vi "运维调试_采配水.vi"() -> ()   [LabVIEW 2016, in "PLC.lvlib"]
uses:
  PLC.lvlib
  <vilib>/Plasmionique/MB Master/MB_Master/MB_Master.lvclass
  <vilib>/Utility/miscctls.llb/LVPointTypeDef.ctl
  <vilib>/Plasmionique/MB Master/MB_Master_TCP/MB_Master_TCP.lvclass
  D:/Program Files (x86)/National Instruments/LabVIEW 2016/vi.lib/Plasmionique/MB Master/MB_Master/MB_Master.lvclass
  <vilib>/NI/Modbus Library/API/Wrapper/Create TCP Slave.vi
  <vilib>/NI/Modbus Library/API/slave/Modbus Slave.lvclass
  <vilib>/Plasmionique/MB Master/MB Master.lvlib
  <vilib>/NI/Modbus Library/API/Wrapper/API Main.lvlib
panel:
  out "R116":i16 caption="储水时间设定"
  out "R115":i16 caption="清洗频次设定"
  out "R114":i16 caption="排液时间"
  out "R113":i16 caption="沉淀池清洗时间"
  out "R112":i16 caption="流通池清洗时间"
  out "R111":i16 caption="吹气时间"
  out "R110":i16 caption="外部管路清洗时间"
  out "R109":i16 caption="配水时间"
  out "R108":i16 caption="沉淀时间"
  out "R107":i16 caption="液位开关报警时间"
  out "R106":i16 caption="进样超时时间"
  out "R105":i16 caption="沉淀池润洗时间"
  out "R104":i16 caption="流通池润洗时间"
  out "沉淀池进样阀计时":dbl
  out "流通池进样阀计时":dbl
  in  "V3-R":bool
  in  "V3-G":bool
  out "状态":u16[](array[numeric])
  in  "更新程序":bool
  out "清洗次数":u16
  out "当前启动泵号":u16(ring) items=["1号泵", "2号泵"]
  in  "R117":u16(ring) caption="水箱储水水体" items=["自来水", "水样"]
  out "增压泵计时":dbl
  out "M2工作计时":dbl
  out "M1工作计时":dbl
  out "泵2反冲洗阀计时":dbl
  out "泵1反冲洗阀计时":dbl
  out "自来水出水阀计时":dbl
  out "进气阀计时":dbl
  out "流通池排液阀计时":dbl
  out "沉淀池排液阀计时":dbl
  out "沉淀池反冲洗阀计时":dbl
  out "流通池反冲洗阀计时":dbl
  out "泵2进样阀计时":dbl
  out "泵1进样阀计时":dbl
  in  "M3":bool
  in  "V11":bool
  in  "V10":bool
  in  "V2":bool
  in  "V1":bool
  in  "V7":bool
  in  "V6":bool
  out "X2":bool caption="X1"
  out "采配水版本号":string
  out "通讯故障":bool
  in  "R102":u16(ring) caption="采水泵工作模式" items=["泵1单泵单管路", "泵2单泵单管路", "双泵双管路"]
  out "X7":bool caption="烟雾报警_YW"
  out "X6":bool caption="泵2过载报警_KM2"
  out "X5":bool caption="泵1过载报警_KM1"
  out "X4":bool caption="外部电源断电报警_DD1"
  out "X3":bool caption="水浸报警_SJ"
  out "X1":bool
  out "X0":bool caption="流通池液位开关_YE1"
  out "集成报警信息":string
  out "R2":i16
  out "R1":i16
  out "多列列表框":i32(listbox)
  in  "V4":bool
  in  "V5":bool
  in  "V9":bool
  in  "V8":bool
  in  "M2":bool
  in  "M1":bool
  in  "返回":bool
  in  "参数设置":bool
  in  "单步启动":bool
  in  "启动":bool
  in  "停止":bool
  # "流程计时："
  # "s"
  # "沉淀池液位开关_YE2"
  # "进样水流开关_JY"
  # "S"
  # "次"
  # "S"
  # "S"
  # "S"
  # "S"
  # "S"
  # "S"
  # "S"
  # "S"
  # "S"
  # "S"
  # "S"
  # "单步计时："
  # "s"
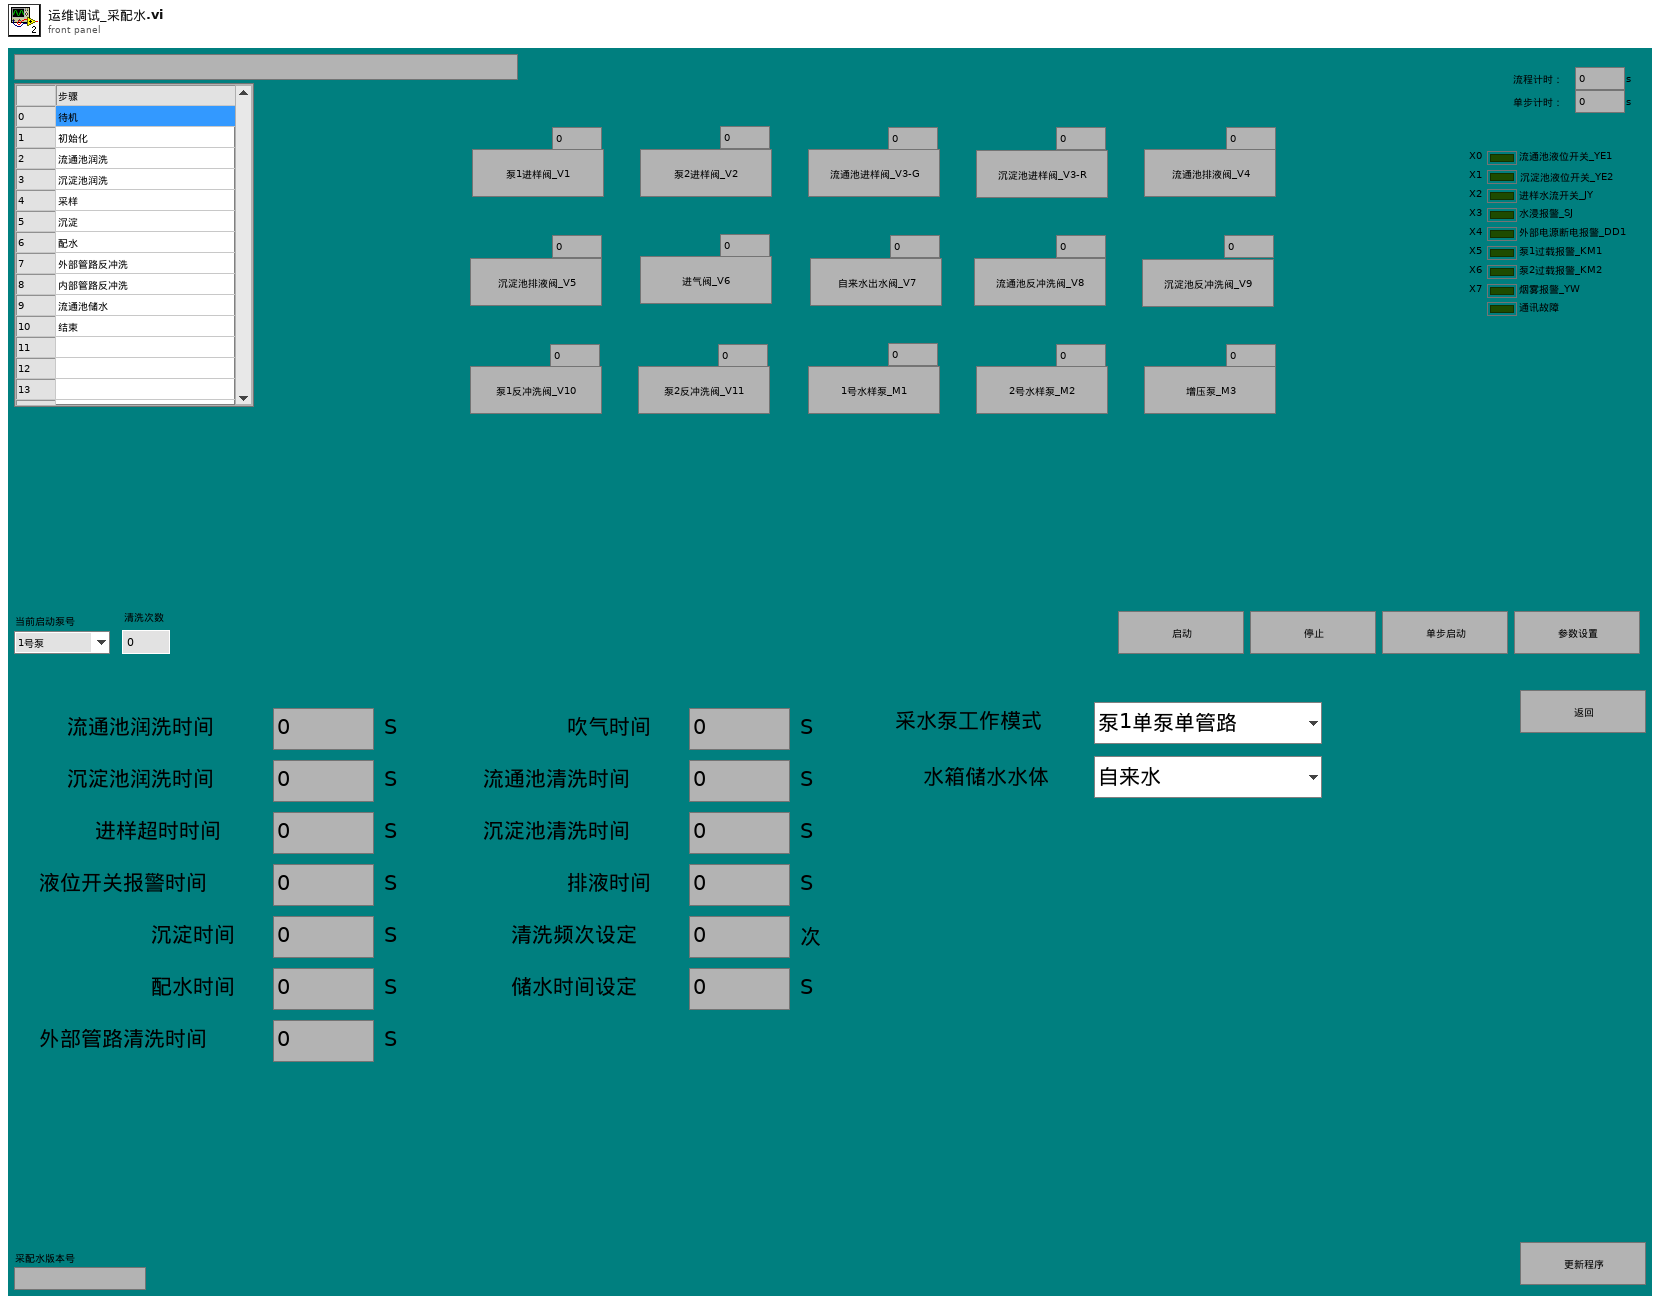
[diagram p1: front panel]
types:
  T1 = cluster{"R100":i16, "R101":i16, "R102":i16, "R103":i16, "R104":i16, "R105":i16, "R106":i16, "R107":i16, "R108":i16, "R109":i16, "R110":i16, "R111":i16, "R112":i16, "R113":i16, "R114":i16, "R115":i16, "R116":i16, "R117":i16, "R118":i16, "R119":i16}
  T2 = cluster{"R200":i16, "R201":i16, "R20 2":i16, "R20 3":i16, "R20 4":i16, "R20 5":i16, "R20 6":i16, "R20 7":i16, "R20 8":i16, "R20 9":i16, "R210":i16, "R211":i16, "R21 2":i16, "R21 3":i16, "R21 4":i16, "R21 5":i16, "R21 6":i16, "R21 7":i16, "R21 8":i16, "R21 9":i16, "R220":i16, "R221":i16, "R22 2":i16, "R22 3":i16}
  T3 = typedef "LVPointTypeDef.ctl" = cluster{"Horizontal":i16, "Vertical":i16}
  T4 = cluster{"时间标识":timestamp, "设备":string, "日志信息":string}
  T5 = cluster{"R0":i16, "R1":i16, "R2":i16, "R3":i16, "R4":i16, "R5":i16, "R6":i16, "R7":i16, "R8":i16, "R9":i16, "R10":i16, "R11":i16, "R12":i16, "R13":i16, "R14":i16, "R15":i16, "R16":i16, "R17":i16, "R18":i16, "R19":i16, "R20":i16, "R21":i16, "R22":i16, "R23":i16, "R24":i16, "R25":i16, "R26":i16, "R27":i16, "R28":i16, "R29":i16, "R30":i16, "R31":i16, "R32":i16, "R33":i16, "R34":i16, "R35":i16, "R36":i16, "R37":i16, "R38":i16, "R39":i16}
  T6 = cluster{"seconds since 1Jan1904":timestamp, "table输入":string, string, "table输入":string}
  T7 = cluster{"时间标识":timestamp, "设备":string, "日志信息":string, "流程参数":string}
  T8 = cluster{"命令":string, cluster{"starting address":u16, "holding register value":u16}}
  T9 = cluster{"命令":string, "数据":cluster{"starting address":u16, "holding register value":u16}}
  T10 = cluster{"命令":string, "数据":cluster{"starting address":u16, "holding register values":u16[]}}
  T11 = cluster{"命令":string, "data":cluster{"starting address":u16, "coil values":bool[]}}
  T12 = cluster{"测试模式":enum16{"正常测试", "集成干预"}, "参数启用":cluster{"氨氮":bool, "总磷":bool, "总氮":bool, "多参数":bool, "CODMn":bool, "CODcr":bool}}
  T13 = enum32{"Bad", "Idle", "Run top level", "Running"}
  T14 = cluster{"starting address":u16, "holding register values":u16[]}
  T15 = cluster{"starting address":u16, "holding register value":u16}
  T16 = cluster{"starting address":u16, "coil values":bool[]}
  T17 = cluster{"Registers[0]":u16, "Registers[1]":u16, "Registers[2]":u16, "Registers[3]":u16, "Registers[4]":u16, "Registers[5]":u16, "Registers[6]":u16, "Registers[7]":u16, "Registers[8]":u16, "Registers[9]":u16, "Registers[10]":u16, "Registers[11]":u16, "Registers[12]":u16, "Registers[13]":u16, "Registers[14]":u16, "Registers[15]":u16, "Registers[16]":u16, "Registers[17]":u16, "Registers[18]":u16, "Registers[19]":u16, "Registers[20]":u16, "Registers[21]":u16, "Registers[22]":u16, "Registers[23]":u16, "Registers[24]":u16, "Registers[25]":u16, "Registers[26]":u16, "Registers[27]":u16, "Registers[28]":u16, "Registers[29]":u16, "Registers[30]":u16, "Registers[31]":u16, "Registers[32]":u16, "Registers[33]":u16, "Registers[34]":u16, "Registers[35]":u16, "Registers[36]":u16, "Registers[37]":u16, "Registers[38]":u16, "Registers[39]":u16}
  T18 = cluster{"Registers[0]":u16, "Registers[1]":u16, "Registers[2]":u16, "Registers[3]":u16, "Registers[4]":u16, "Registers[5]":u16, "Registers[6]":u16, "Registers[7]":u16, "Registers[8]":u16, "Registers[9]":u16, "Registers[10]":u16, "Registers[11]":u16, "Registers[12]":u16, "Registers[13]":u16, "Registers[14]":u16, "Registers[15]":u16, "Registers[16]":u16, "Registers[17]":u16, "Registers[18]":u16, "Registers[19]":u16, "Registers[20]":u16, "Registers[21]":u16, "Registers[22]":u16, "Registers[23]":u16}
  T19 = cluster{"Registers[0]":u16, "Registers[1]":u16, "Registers[2]":u16, "Registers[3]":u16, "Registers[4]":u16, "Registers[5]":u16}
  T20 = cluster{"Registers[0]":u16, "Registers[1]":u16, "Registers[2]":u16, "Registers[3]":u16, "Registers[4]":u16, "Registers[5]":u16, "Registers[6]":u16, "Registers[7]":u16, "Registers[8]":u16, "Registers[9]":u16, "Registers[10]":u16, "Registers[11]":u16, "Registers[12]":u16, "Registers[13]":u16, "Registers[14]":u16, "Registers[15]":u16, "Registers[16]":u16, "Registers[17]":u16, "Registers[18]":u16, "Registers[19]":u16}
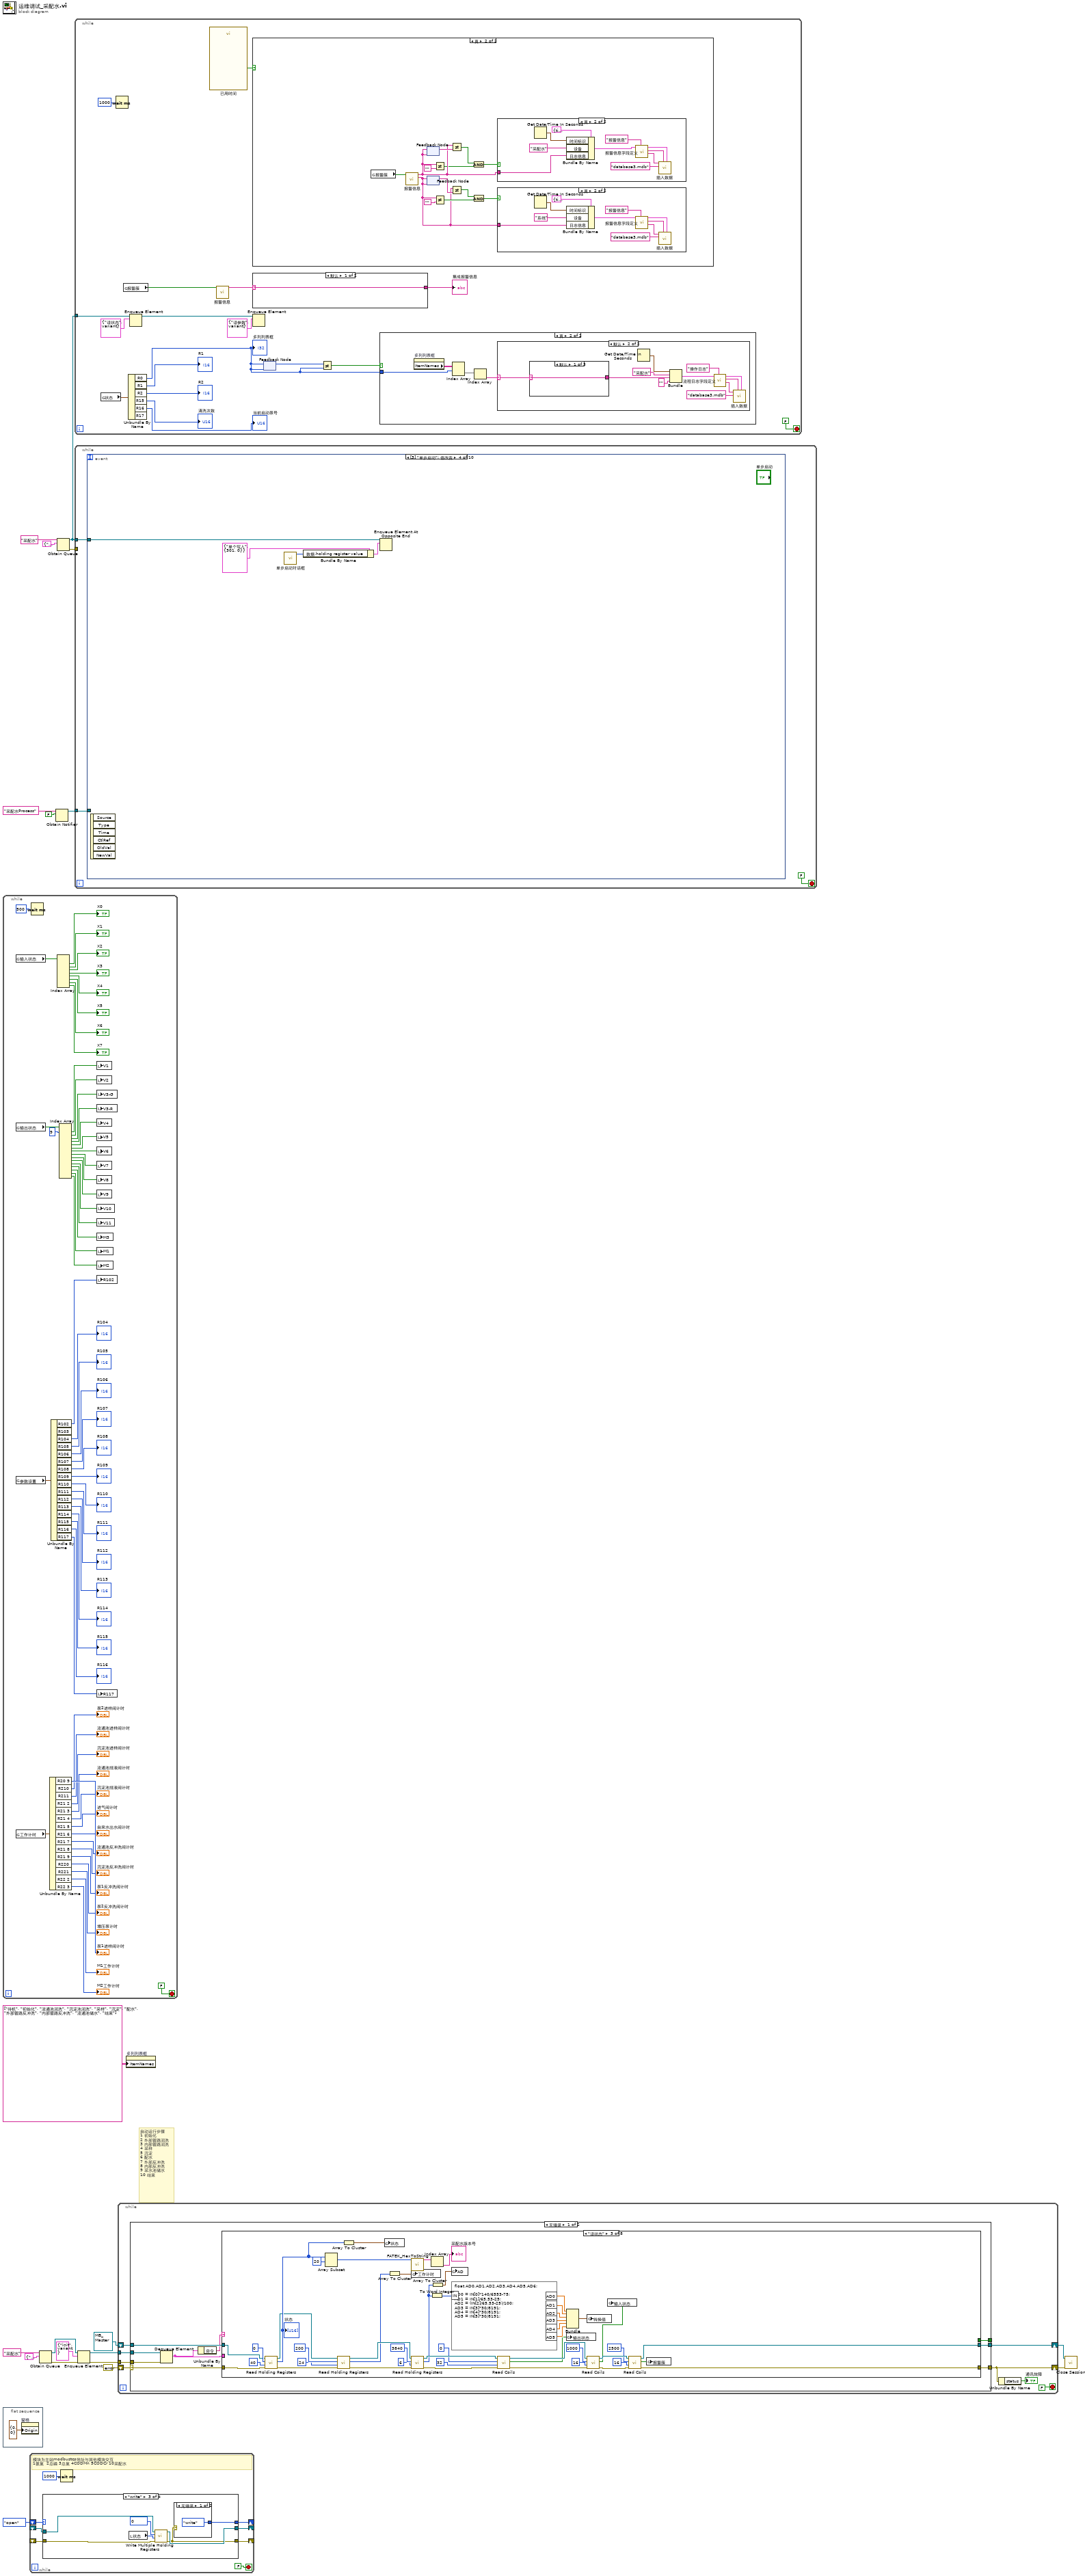
[diagram p0: block diagram]
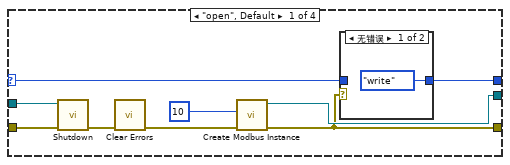
[diagram p2: hidden frame]
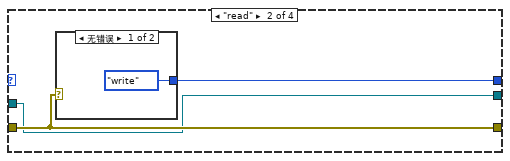
[diagram p4: hidden frame]
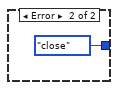
[diagram p5: hidden frame]
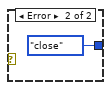
[diagram p6: hidden frame]
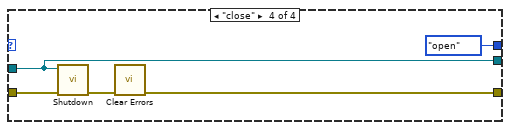
[diagram p7: hidden frame]
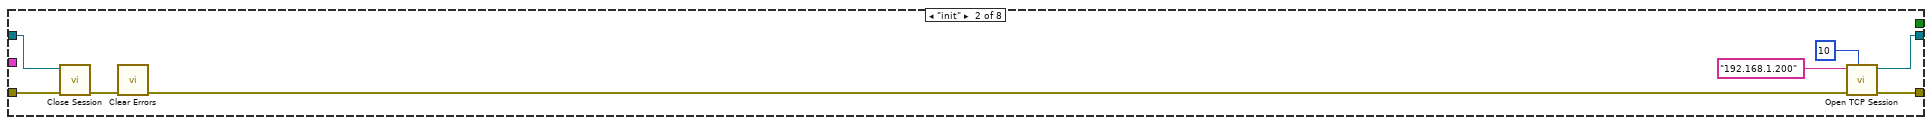
[diagram p9: hidden frame]
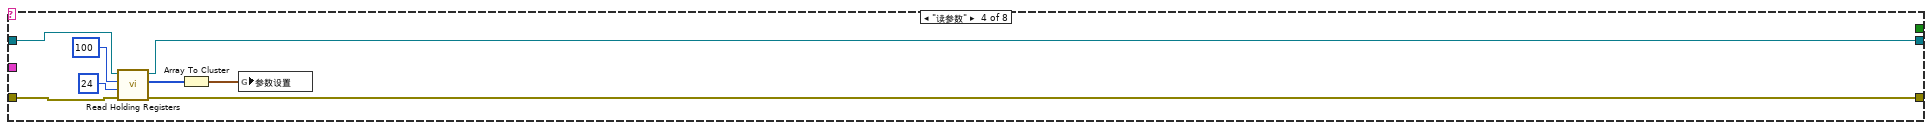
[diagram p10: hidden frame]
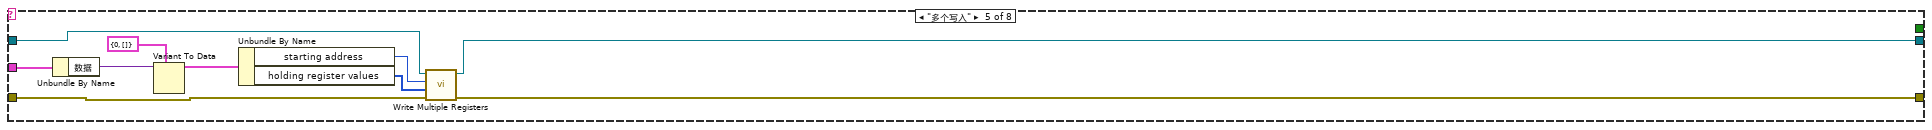
[diagram p11: hidden frame]
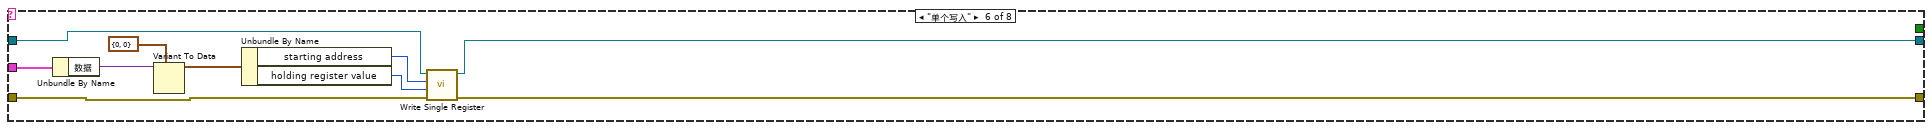
[diagram p12: hidden frame]
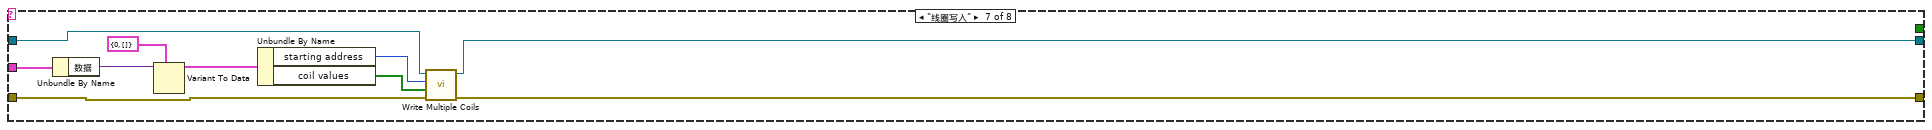
[diagram p13: hidden frame]
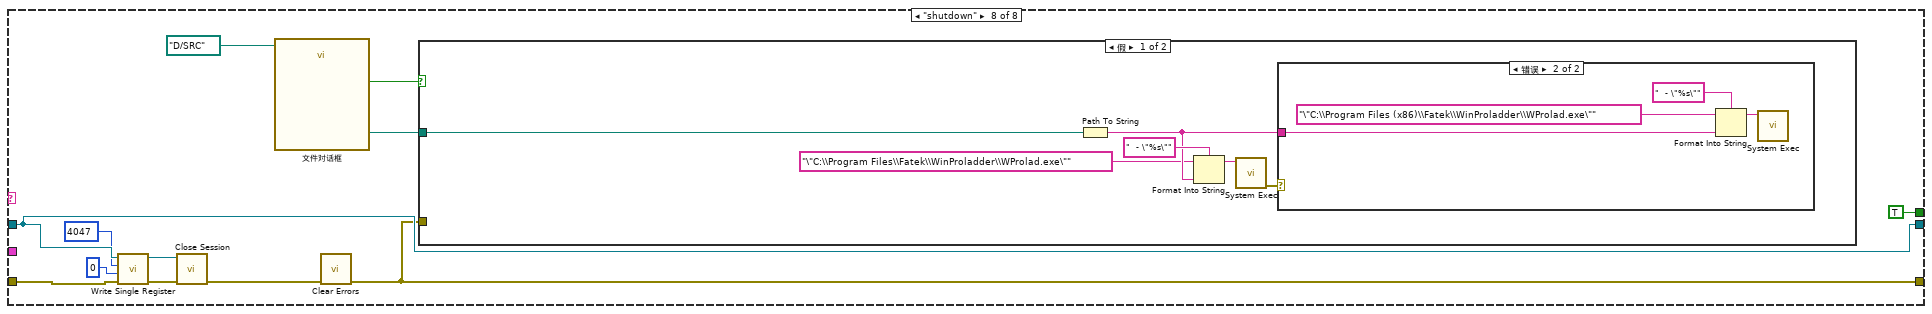
[diagram p14: hidden frame]
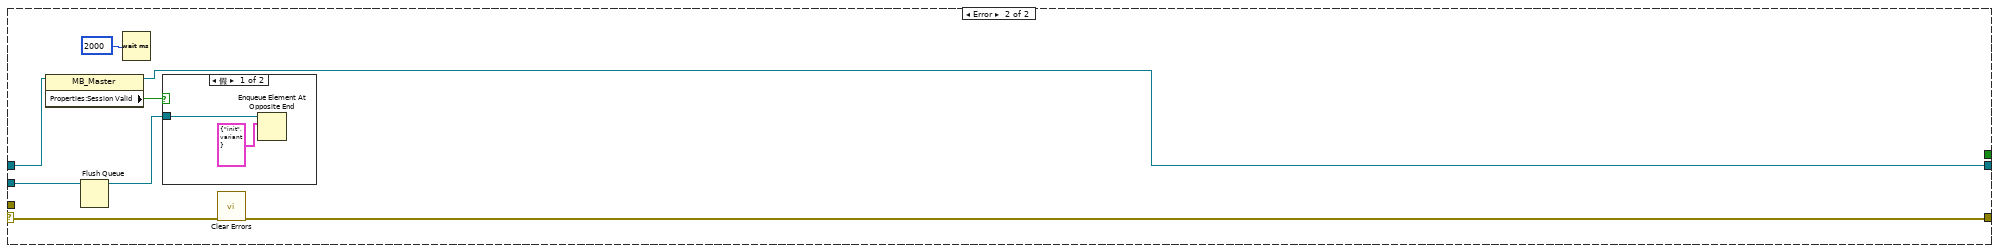
[diagram p17: hidden frame]
diagram:
  # "自动运行步骤\n1 初始化\n2 外部管路润洗\n3 内部管路润洗\n4 采样\n5 沉淀\n6 配水\n7 外部反冲洗\n8 内部反冲洗\n9 采水池储水\n10 结束"
  n1 = while {
    stop <- FALSE stop-if-true
    n2 = global read "采配水全局变量.vi" "输入状态"() -> (w63:bool[])
    n3 = global read "采配水全局变量.vi" "输出状态"() -> (w79:bool[])
    n4 = global read "采配水全局变量.vi" "参数设置"() -> (w36:T1)
    n5 = global read "采配水全局变量.vi" "工作计时"() -> (w52:T2)
    n6 = Wait (ms)(milliseconds to wait=u32 500 ("等待时间（毫秒）")) -> ()  [unwired: 1 out]
    n7 = Unbundle By Name(w52) -> ("R20 9"=→"泵1进样阀计时":i16, "R210"=→"泵2进样阀计时":i16, "R211"=→"流通池进样阀计时":i16, "R21 2"=→"沉淀池进样阀计时":i16, "R21 3"=→"流通池排液阀计时":i16, "R21 4"=→"沉淀池排液阀计时":i16, "R21 5"=→"进气阀计时":i16, "R21 6"=→"自来水出水阀计时":i16, "R21 7"=→"流通池反冲洗阀计时":i16, "R21 8"=→"沉淀池反冲洗阀计时":i16, "R21 9"=→"泵1反冲洗阀计时":i16, "R220"=→"泵2反冲洗阀计时":i16, "R221"=→"增压泵计时":i16, "R22 2"=→"M1工作计时":i16, "R22 3"=→"M2工作计时":i16)
    n8 = Unbundle By Name(w36) -> ("R102"=w35:i16, "R104"=→"R104":i16, "R105"=→"R105":i16, "R106"=→"R106":i16, "R107"=→"R107":i16, "R108"=→"R108":i16, "R109"=→"R109":i16, "R110"=→"R110":i16, "R111"=→"R111":i16, "R112"=→"R112":i16, "R113"=→"R113":i16, "R114"=→"R114":i16, "R115"=→"R115":i16, "R116"=→"R116":i16, "R117"=w21:i16)  [unwired: 1 out]
    n9 = Index Array(array=w63) -> (element #1=→"X0":bool, element #2=→"X1":bool, element #3=→"X2":bool, element #4=→"X3":bool, element #5=→"X4":bool, element #6=→"X5":bool, element #7=→"X6":bool, element #8=→"X7":bool)  [unwired: 8 in]
    n10 = Index Array(array=w79, index #1=9 ("索引")) -> (element #1=w77:bool, element #2=w76:bool, element #3=w75:bool, element #4=w74:bool, element #5=w73:bool, element #6=w72:bool, element #7=w71:bool, element #8=w70:bool, element #9=w53:bool, element #10=w54:bool, element #11=w69:bool, element #12=w68:bool, element #13=w67:bool, element #14=w66:bool, element #15=w65:bool)  [unwired: 14 in]
    n11 = local write "V1"(w77) -> ()
    n12 = local write "V2"(w76) -> ()
    n13 = local write "V3-G"(w75) -> ()
    n14 = local write "V3-R"(w74) -> ()
    n15 = local write "V4"(w73) -> ()
    n16 = local write "V5"(w72) -> ()
    n17 = local write "V6"(w71) -> ()
    n18 = local write "V7"(w70) -> ()
    n19 = local write "V8"(w53) -> ()
    n20 = local write "V9"(w54) -> ()
    n21 = local write "V10"(w69) -> ()
    n22 = local write "V11"(w68) -> ()
    n23 = local write "M3"(w67) -> ()
    n24 = local write "M1"(w66) -> ()
    n25 = local write "M2"(w65) -> ()
    n26 = local write "R102"(w35) -> ()
    n27 = local write "R117"(w21) -> ()
  }
  n28 = flat-sequence {
    frame #0 {
      n29 = property on="窗格" class="Pane"("Origin"=T3 {"Horizontal"=0, "Vertical"=0} ("原点")) -> ()  [unwired: 2 in, 2 out]
    }
  }
  n30 = while {
    shift-right: [w87] -> _
    shift-left: _ -> [w89]
    shift-right: [w86] -> _
    shift-left: _ -> [w88]
    shift-right: [w83] -> _
    shift-left: enum16{"open", "read", "write", "close"}."open" -> [w84]
    stop <- FALSE stop-if-true
    # "模块为主站modbustcp地址与其他模块交互\n1氨氮  2总磷 3总氮 4CODMn 5CODCr 10采配水"
    n31 = case shown="\"write\"" w84 {
      selector: w84 -> [w98 _ _ _]
      tunnel: w89 -> [w92 w101 w111 w117]
      tunnel: w88 -> [w91 w102 w110 w116]
      tunnel: [w95 w101 w108 w117] -> w87
      tunnel: [w94 w102 w107 w119] -> w86
      tunnel: [w97 w103 w112 enum16{"open", "read", "write", "close"}."open"] -> w83
      frame "open", Default {
        n32 = call-dynamic "Shutdown.vi"("error in"=w91, "Modbus slave in"=w92) -> ("error out"=w90:errorcluster)  [unwired: 9 in]
        n33 = call <vilib>:"Clear Errors.vi"("error in (no error)"=w90) -> ("error out"=w93:errorcluster)  [unwired: 5 in, 1 out]
        n34 = call-poly <vilib>:"Create Modbus Instance.vi"("error in"=w93, "port (502)"=u16 10) -> ("error out"=w94:errorcluster, "TCP slave instance"=w95:refnum<class "Modbus Slave.lvclass">)  [unwired: 8 in]
        n35 = case shown="无错误" w94 {
          tunnel: w98 -> [_ w100]
          tunnel: [enum16{"open", "read", "write", "close"}."write" w100] -> w97
          frame No Error {
          }
          frame Error {
          }
        }
      }
      frame "read" {
        n36 = case shown="无错误" w102 {
          tunnel: [enum16{"open", "read", "write", "close"}."write" enum16{"open", "read", "write", "close"}."close"] -> w103
          frame No Error {
          }
          frame Error {
          }
        }
      }
      frame "write" {
        n37 = local read "状态"() -> (w106:u16[])
        n38 = call-dynamic "Write Multiple Holding Registers.vi"("error in"=w110, "registers to write"=w106, "starting address"=u16 0, "Modbus slave in"=w111) -> ("error out"=w107:errorcluster, "Modbus slave out"=w108:refnum<class "Modbus Slave.lvclass">)  [unwired: 6 in]
        n39 = case shown="无错误" w107 {
          tunnel: [enum16{"open", "read", "write", "close"}."write" enum16{"open", "read", "write", "close"}."close"] -> w112
          frame No Error {
          }
          frame Error {
          }
        }
      }
      frame "close" {
        n40 = call-dynamic "Shutdown.vi"("error in"=w116, "Modbus slave in"=w117) -> ("error out"=w115:errorcluster)  [unwired: 9 in]
        n41 = call <vilib>:"Clear Errors.vi"("error in (no error)"=w115) -> ("error out"=w119:errorcluster)  [unwired: 5 in, 1 out]
      }
    }
    n42 = Wait (ms)(milliseconds to wait=u32 1000 ("等待时间（毫秒）")) -> ()  [unwired: 1 out]
  }
  n43 = Obtain Queue(name (unnamed)="采配水" ("名称（未命名）"), element data type=cluster{"命令":string, "数据":variant} {"命令"="", "数据"=variant}) -> (queue out=w10:refnum<queue>, error out=w9:errorcluster)  [unwired: 3 in, 1 out]
  n44 = Obtain Notifier(name (unnamed)="采配水Process" ("名称（未命名）"), notification data type=FALSE) -> (notifier out=w13:refnum<notifier>)  [unwired: 2 in, 2 out]
  n45 = Obtain Queue(name (unnamed)="采配水" ("名称（未命名）"), element data type=cluster{"命令":string, "数据":variant} {"命令"="", "数据"=variant}) -> (queue out=w17:refnum<queue>, error out=w18:errorcluster)  [unwired: 3 in, 1 out]
  n46 = while {
    tunnel: w17 -> [w136]
    stop <- FALSE stop-if-true
    n47 = global read "采配水全局变量.vi" "状态"() -> (w134:T5)
    n48 = Wait (ms)(milliseconds to wait=u32 1000 ("等待时间（毫秒）")) -> ()  [unwired: 1 out]
    n49 = global read "采配水全局变量.vi" "报警簇"() -> (w130:bool[])
    n50 = Unbundle By Name(w134) -> ("R0"=w123:i16, "R1"=→"R1":i16, "R2"=→"R2":i16, "R15"=→"清洗次数":i16, "R16"=→"当前启动泵号":i16)  [unwired: 1 out]
    "多列列表框" <- w123
    n51 = Enqueue Element(queue=w136, element=cluster{"命令":string, "数据":variant} {"命令"="读状态", "数据"=variant} ("元素")) -> (queue out=w125:refnum<queue>)  [unwired: 2 in, 2 out]
    n52 = call "已用时间"() -> ("Time has Elapsed"=w128:bool)  [unwired: 12 in, 7 out]
    n53 = call "报警信息.vi"("报警簇"=w130) -> ("采配水报警信息"=w122:string)  [unwired: 9 in, 1 out]
    n54 = case shown="真" w128 {
      frame False {
      }
      frame True {
        n55 = global read "采配水全局变量.vi" "报警簇"() -> (w150:bool[])
        n56 = call "报警信息.vi"("报警簇"=w150) -> ("系统报警信息"=w139:string, "采配水报警信息"=w146:string)  [unwired: 9 in]
        n57 = feedback #1(w146) -> (w149:string)
        n58 = feedback-in #1(w146) -> ()
        n59 = feedback #2(w139) -> (w140:string)
        n60 = feedback-in #2(w139) -> ()
        n61 = Not Equal?(x=w146, y="") -> (x != y?=w144:bool)
        n62 = Not Equal?(x=w139, y="") -> (x != y?=w143:bool)
        n63 = Not Equal?(x=w146, y=w149) -> (x != y?=w148:bool)
        n64 = Not Equal?(x=w139, y=w140) -> (x != y?=w141:bool)
        n65 = And(x=w148, y=w144) -> (x .and. y?=w147:bool)
        n66 = And(x=w141, y=w143) -> (x .and. y?=w138:bool)
        n67 = case shown="真" w147 {
          tunnel: w146 -> [_ w161]
          frame False {
          }
          frame True {
            n68 = Get Date/Time In Seconds() -> (seconds since 1Jan1904=w163:timestamp)
            n69 = Bundle By Name(cluster=T4 {"时间标识"=timestamp(0 s since 1904-01-01), "设备"="", "日志信息"=""} ("data in"), "时间标识"=w163, "设备"="采配水", "日志信息"=w161) -> (w164:T4)
            n70 = call "报警信息字段定义.vi"("table输入"="报警信息", "data in"=w164) -> ("table输出"=w168:string, "columns"=w169:string[], "data out"=w170:T4)  [unwired: 7 in]
            n71 = call "插入数据.vi"("data"=w170, "columns"=w169, "database"="database3.mdb", "table"=w168) -> ()  [unwired: 7 in, 1 out]
          }
        }
        n72 = case shown="真" w138 {
          tunnel: w139 -> [_ w151]
          frame False {
          }
          frame True {
            n73 = Get Date/Time In Seconds() -> (seconds since 1Jan1904=w153:timestamp)
            n74 = Bundle By Name(cluster=T4 {"时间标识"=timestamp(0 s since 1904-01-01), "设备"="", "日志信息"=""} ("data in"), "时间标识"=w153, "设备"="系统", "日志信息"=w151) -> (w154:T4)
            n75 = call "报警信息字段定义.vi"("table输入"="报警信息", "data in"=w154) -> ("table输出"=w158:string, "columns"=w159:string[], "data out"=w160:T4)  [unwired: 7 in]
            n76 = call "插入数据.vi"("data"=w160, "columns"=w159, "database"="database3.mdb", "table"=w158) -> ()  [unwired: 7 in, 1 out]
          }
        }
      }
    }
    n77 = case shown="默认" w122 {
      selector: w122 -> [w171 _]
      tunnel: [w171 w172] -> w129
      frame Default {
      }
      frame "" {
        n78 = global read "采配水全局变量.vi" "运行状态显示"() -> (w172:string)
      }
    }
    "集成报警信息" <- w129
    n79 = Enqueue Element(queue=w125, element=cluster{"命令":string, "数据":variant} {"命令"="读参数", "数据"=variant} ("元素")) -> ()  [unwired: 2 in, 3 out]
    n80 = feedback-in #3(w123) -> ()
    n81 = feedback #3(w123) -> (w124:i16)
    n82 = Not Equal?(x=w124, y=w123) -> (x != y?=w131:bool)
    n83 = case shown="真" w131 {
      tunnel: w123 -> [_ w175]
      frame False {
      }
      frame True {
        n84 = property on="多列列表框" class="MCListbox (严格)"() -> ("ItemNames"=w176:string[][])  [unwired: 2 in, 2 out]
        n85 = Index Array(array=w176, index (row)=w175) -> (element=w174:string[])  [unwired: 1 in]
        n86 = Index Array(array=w174) -> (element=w173:string)  [unwired: 1 in]
        n87 = case shown="默认" w173 {
          selector: w173 -> [_ w178]
          frame "待机" {
          }
          frame Default {
            n88 = case shown="默认" w178 {
              selector: w178 -> [w188 _ _]
              tunnel: [w188 "-->>启动" "-->>结束"] -> w177
              frame Default {
              }
              frame "初始化" {
              }
              frame "结束" {
              }
            }
            n89 = Get Date/Time In Seconds() -> (seconds since 1Jan1904=w182:timestamp)
            n90 = Bundle("seconds since 1Jan1904"=w182, "table输入"="采配水", w177, "table输入"="") -> (w180:T6)  [unwired: 1 in]
            n91 = call "流程日志字段定义.vi"("table输入"="操作日志", "data in"=w180) -> ("table输出"=w185:string, "columns"=w186:string[], "data out"=w187:T7)  [unwired: 7 in]
            n92 = call "插入数据.vi"("data"=w187, "columns"=w186, "database"="database3.mdb", "table"=w185) -> ()  [unwired: 7 in, 1 out]
          }
        }
      }
    }
  }
  n93 = while {
    tunnel: w17 -> [w192]
    tunnel: w18 -> [_]
    tunnel: w13 -> [w191]
    stop <- FALSE stop-if-true
    n94 = event shown="[3] \"单步启动\": 值改变" {
      selector: _ -> [_ _ _ _ _ _ _ _ _ _]
      dyn-events: _ -> [_ _ _ _ _ _ _ _ _ _]
      timeout: _ -> [_ _ _ _ _ _ _ _ _ _]
      tunnel: w192 -> [_ w196 w199 w221 w242 _ _ _ w267 w271]
      tunnel: w191 -> [_ w195 w198 _ _ _ _ _ _ _]
      event Timeout {
        n95 = event-data() -> ()  [unwired: 1 in, 3 out]
      }
      event "停止": Value Change {
        n96 = event-data() -> ()  [unwired: 1 in, 6 out]
        n97 = Send Notification(notification=TRUE ("通知"), notifier=w195) -> ()  [unwired: 1 in, 2 out]
        n98 = Enqueue Element At Opposite End(queue=w196, element=T8 {"命令"="单个写入", {"starting address"=300, "holding register value"=2}} ("元素")) -> ()  [unwired: 2 in, 3 out]
      }
      event "启动": Value Change {
        n99 = event-data() -> ()  [unwired: 1 in, 6 out]
        n100 = disable-structure shown="禁用" {
          disable-tunnel: w199 -> [w217 _]
          frame Disabled {
            n101 = Enqueue Element At Opposite End(queue=w217, element=T8 {"命令"="单个写入", {"starting address"=300, "holding register value"=1}} ("元素")) -> ()  [unwired: 2 in, 3 out]
          }
          frame Enabled {
          }
        }
        n102 = flat-sequence {
          tunnel: w198 -> [w200]
          frame #0 {
            n103 = Cancel Notification(0:w200) -> ()  [unwired: 1 in, 3 out]
          }
          frame #1 {
            n104 = call "手动启动选择对话框.vi"() -> ("确定"=w202:bool, "输出簇"=w201:T12)  [unwired: 10 in]
            n105 = case shown="真" w202 {
              tunnel: w201 -> [_ w203]
              frame False {
              }
              frame True {
                n106 = vi-ref "PLC.lvlib:一体站流程自动启动.vi"() -> (w206:refnum<vi>)
                n107 = property class="VI"(reference=w206) -> ("Name"=w205:string, "Exec.State"=w204:T13)  [unwired: 1 in, 2 out]
                n108 = case shown="\"Idle\"" w204 {
                  tunnel: w205 -> [_ w214 _ _]
                  tunnel: w203 -> [_ w207 _ _]
                  frame "Bad", Default {
                  }
                  frame "Idle" {
                    n109 = Open VI Reference(type specifier VI Refnum (for type only)=refnum<vi> refnum, vi path=w214, options=128 ("选项")) -> (vi reference=w212:refnum<vi>, error out=w210:errorcluster)  [unwired: 3 in]
                    n110 = call-by-ref "开始异步调用"(reference=w212, error in=w210, "参数"=w207) -> (reference out=w211:refnum<vi>, error out=w209:errorcluster)  [unwired: 11 in]
                    n111 = Close Reference(reference=w211, error in (no error)=w209) -> ()  [unwired: 1 out]
                  }
                  frame "Run top level" {
                  }
                  frame "Running" {
                    n112 = One Button Dialog(message="流程已启动，无需重复启动！" ("消息")) -> ()  [unwired: 1 in, 1 out]
                  }
                }
              }
            }
          }
        }
      }
      event "单步启动": Value Change {
        n113 = event-data() -> ()  [unwired: 1 in, 6 out]
        n114 = call "单步启动对话框.vi"() -> ("单步启动步骤输出"=w218:u16)  [unwired: 11 in]
        n115 = Bundle By Name(cluster=T9 {"命令"="单个写入", "数据"={"starting address"=301, "holding register value"=0}} ("元素"), "数据.holding register value"=w218) -> (w219:T9)
        n116 = Enqueue Element At Opposite End(queue=w221, element=w219) -> ()  [unwired: 2 in, 3 out]
      }
      event "R104", "R117", "R105", "R106", "R107", "R108", "R109", "R110", "R111", "R112", "R113", "R114", "R115", "R116", "R102": Value Change {
        n117 = event-data() -> ()  [unwired: 1 in, 6 out]
        n118 = local read "R104"() -> (w236:i16)
        n119 = local read "R105"() -> (w235:i16)
        n120 = local read "R106"() -> (w234:i16)
        n121 = local read "R107"() -> (w233:i16)
        n122 = local read "R108"() -> (w232:i16)
        n123 = local read "R109"() -> (w231:i16)
        n124 = local read "R110"() -> (w230:i16)
        n125 = local read "R111"() -> (w229:i16)
        n126 = local read "R112"() -> (w228:i16)
        n127 = local read "R113"() -> (w227:i16)
        n128 = local read "R114"() -> (w226:i16)
        n129 = local read "R115"() -> (w225:i16)
        n130 = local read "R116"() -> (w224:i16)
        n131 = Build Array("R102", u16 0 ("元素"), w236, w235, w234, w233, w232, w231, w230, w229, w228, w227, w226, w225, w224, "R117") -> (w237:u16[])
        n132 = Bundle By Name(cluster=T10 {"命令"="多个写入", "数据"={"starting address"=0, "holding register values"=[]}} ("元素"), "数据.starting address"=u16 102, "数据.holding register values"=w237) -> (w239:T10)
        n133 = Enqueue Element At Opposite End(queue=w242, element=w239) -> ()  [unwired: 2 in, 3 out]
      }
      event "R104", "R105", "R106", "R107", "R108", "R109", "R110", "R111", "R112", "R113", "R114", "R115", "R116": Mouse Down {
        n134 = event-data() -> ("CtlRef"=w246:refnum<vi>)  [unwired: 1 in, 7 out]
        n135 = property class="DigNum (严格)"(reference=w246) -> (reference out=w244:refnum<vi>, "Value"=w245:i16)  [unwired: 1 in, 1 out]
        n136 = call "数字键盘.vi"("OldNumber"=w245) -> ("NewNumber"=w243:sgl)
        n137 = property class="DigNum (严格)"(reference=w244, "Val(Sgnl)"=w243) -> ()  [unwired: 1 in, 2 out]
      }
      event "参数设置": Value Change {
        n138 = event-data() -> ()  [unwired: 1 in, 6 out]
        n139 = property on="窗格" class="Pane"("Origin"=T3 {"Horizontal"=0, "Vertical"=628} ("原点")) -> ()  [unwired: 2 in, 2 out]
      }
      event "返回": Value Change {
        n140 = event-data() -> ()  [unwired: 1 in, 6 out]
        n141 = property on="窗格" class="Pane"("Origin"=T3 {"Horizontal"=0, "Vertical"=0} ("原点")) -> ()  [unwired: 2 in, 2 out]
      }
      event "M1", "M2", "V8", "V9", "V5", "V4", "V6", "V7", "V1", "V2", "V10", "V11", "M3", "V3-G", "V3-R": Value Change {
        n142 = event-data() -> ()  [unwired: 1 in, 6 out]
        n143 = Build Array("V1", "V2", "V3-G", "V3-R", "V4", "V5", "V6", "V7", "V8", "V9", "V10", "V11", "M3", "M1", "M2") -> (w264:bool[])
        n144 = Bundle By Name(cluster=T11 {"命令"="线圈写入", "data"={"starting address"=2409, "coil values"=[]}} ("元素"), "data.coil values"=w264) -> (w265:T11)
        n145 = Enqueue Element(queue=w267, element=w265) -> ()  [unwired: 2 in, 3 out]
      }
      event "更新程序": Value Change {
        n146 = event-data() -> ("NewVal"=w268:bool)  [unwired: 1 in, 5 out]
        n147 = case shown="真" w268 {
          tunnel: [cluster{"命令":string, "数据":variant} {"命令"="init", "数据"=variant} ("元素") w275] -> w270
          frame False {
          }
          frame True {
            n148 = Two Button Dialog(message="警告，非专业人士请勿进行此操作！！！\n请确认是否继续？" ("消息")) -> (T button?=w274:bool)  [unwired: 2 in]
            n149 = case shown="真" w274 {
              tunnel: [_ cluster{"命令":string, "数据":variant} {"命令"="shutdown", "数据"=variant} ("元素")] -> w275
              frame False {
                n150 = local write "更新程序"(FALSE ("释放串口")) -> ()
              }
              frame True {
              }
            }
          }
        }
        n151 = Flush Queue(queue=w271) -> (queue out=w269:refnum<queue>)  [unwired: 1 in, 2 out]
        n152 = Enqueue Element(queue=w269, element=w270) -> ()  [unwired: 2 in, 3 out]
      }
    }
  }
  n153 = Enqueue Element(queue=w10, element=cluster{"命令":string, "数据":variant} {"命令"="init", "数据"=variant} ("元素"), error in (no error)=w9) -> (queue out=w5:refnum<queue>, error out=w7:errorcluster)  [unwired: 1 in, 1 out]
  n154 = while {
    tunnel: w5 -> [w282]
    tunnel: w7 -> [w281]
    shift-right: [w285] -> w4
    shift-left: refnum<class "MB_Master.lvclass"> refnum ("MB session out") -> [w284]
    shift-right: [w278] -> w1
    shift-left: errorcluster {"status"=FALSE, "code"=0, "source"=""} ("error out") -> [w283]
    stop <- FALSE stop-if-true
    n155 = case shown="无错误" w283 {
      selector: w283 -> [w291 w415]
      tunnel: [w294 w412] -> w285
      tunnel: w284 -> [w293 w413]
      tunnel: [w292 w416] -> w278
      tunnel: w282 -> [w288 w419]
      tunnel: w281 -> [w287 _]
      tunnel: [w289 _] -> _
      frame No Error {
        n156 = Dequeue Element(queue=w288, error in (no error)=w287) -> (element=w286:cluster{"命令":string, "数据":variant})  [unwired: 1 in, 3 out]
        n157 = Unbundle By Name(w286) -> ("命令"=w290:string)
        n158 = case shown="\"读状态\"" w290 {
          tunnel: [w296 w297 w306 w354 w366 w376 w386 w399] -> w294
          tunnel: w293 -> [w296 w302 w341 w359 w369 w379 w389 w399]
          tunnel: [w295 w298 w305 w353 w367 w377 w387 w390] -> w292
          tunnel: w291 -> [w295 w304 w344 w358 w368 w378 w388 w395]
          tunnel: [_ _ _ _ _ _ _ TRUE] -> w289
          tunnel: w286 -> [_ _ _ _ w365 w375 w385 _]
          frame "idle", Default {
          }
          frame "init" {
            n159 = call-dynamic "Close Session.vi"("error in (no error)"=w304, "MB session in"=w302) -> ("error out"=w303:errorcluster)  [unwired: 9 in]
            n160 = call <vilib>:"Clear Errors.vi"("error in (no error)"=w303) -> ("error out"=w299:errorcluster)  [unwired: 5 in, 1 out]
            n161 = call <vilib>:"Open TCP Session.vi"("Slave ID (255)"=u8 10, "error in (no error)"=w299, "IP Address"="192.168.1.200") -> ("error out"=w298:errorcluster, "MB_TCP session"=w297:refnum<class "MB_Master_TCP.lvclass">)  [unwired: 7 in]
          }
          frame "读状态" {
            n162 = call <vilib>:"Read Holding Registers.vi"("error in (no error)"=w344, "quantity"=u16 40 ("number of holding registers"), "starting address"=u16 0, "MB session in"=w341) -> ("error out"=w313:errorcluster, "Registers"=w316:u16[], "MB session out"=w314:refnum<class "MB_Master.lvclass">)  [unwired: 5 in]
            "状态" <- w316
            n163 = Array Subset(array=w316, index=20 ("索引")) -> (w320:u16[])  [unwired: 1 in]
            n164 = call <vilib>:"Read Holding Registers.vi"("error in (no error)"=w313, "quantity"=u16 24, "starting address"=u16 200, "MB session in"=w314) -> ("error out"=w312:errorcluster, "Registers"=w308:u16[], "MB session out"=w311:refnum<class "MB_Master.lvclass">)  [unwired: 5 in]
            n165 = Array To Cluster(array=w316) -> (cluster=w315:T17)
            n166 = global write "采配水全局变量.vi" "状态"(w315) -> ()
            n167 = Array To Cluster(array=w308) -> (cluster=w307:T18)
            n168 = call "FATEK_HexToString.vi"("数组"=w320) -> ("STRING"=w319:string[])  [unwired: 10 in]
            n169 = global write "采配水全局变量.vi" "工作计时"(w307) -> ()
            n170 = call <vilib>:"Read Holding Registers.vi"("error in (no error)"=w312, "quantity"=u16 6 ("number of holding registers"), "starting address"=u16 3840, "MB session in"=w311) -> ("error out"=w337:errorcluster, "Registers"=w323:u16[], "MB session out"=w338:refnum<class "MB_Master.lvclass">)  [unwired: 5 in]
            n171 = Index Array(array=w319) -> (element=→"采配水版本号":string)  [unwired: 1 in]
            n172 = To Word Integer(number=w323) -> (16bit integer=w322:i16[])
            n173 = Array To Cluster(array=w323) -> (cluster=w351:T19)
            n174 = global write "采配水全局变量.vi" "AD"(w351) -> ()
            n175 = formula code="float AD0,AD1,AD2,AD3,AD4,AD5,AD6;\n\nAD0 = IN[0]*140/6553-75;\nAD1 = IN[1]/65.53-25;\nAD2 = (IN[2]/65.53-25)/100;\nAD3 = IN[3]*30/8191;\nAD4 = IN[4]*30/8191;\nAD5 = IN[5]*30/8191;"("IN"=w322) -> ("AD0"=w349:dbl, "AD1"=w348:dbl, "AD2"=w317:dbl, "AD3"=w347:dbl, "AD4"=w346:dbl, "AD5"=w345:dbl)
            n176 = call <vilib>:"Read Coils.vi"("error in (no error)"=w337, "quantity"=u16 32 ("number of coils"), "starting address"=u16 0, "MB session in"=w338) -> ("error out"=w333:errorcluster, "Coils"=w324:bool[], "MB session out"=w334:refnum<class "MB_Master.lvclass">)  [unwired: 5 in]
            n177 = global write "采配水全局变量.vi" "输出状态"(w324) -> ()
            n178 = Bundle(w349, w348, w317, w347, w346, w345) -> (w350:cluster{dbl, dbl, dbl, dbl, dbl, dbl})  [unwired: 1 in]
            n179 = global write "采配水全局变量.vi" "转换值"(w350) -> ()
            n180 = call <vilib>:"Read Coils.vi"("error in (no error)"=w333, "quantity"=u16 16 ("number of coils"), "starting address"=u16 1000, "MB session in"=w334) -> ("error out"=w329:errorcluster, "Coils"=w325:bool[], "MB session out"=w330:refnum<class "MB_Master.lvclass">)  [unwired: 5 in]
            n181 = global write "采配水全局变量.vi" "输入状态"(w325) -> ()
            n182 = call <vilib>:"Read Coils.vi"("error in (no error)"=w329, "quantity"=u16 16 ("number of coils"), "starting address"=u16 2500, "MB session in"=w330) -> ("error out"=w305:errorcluster, "Coils"=w326:bool[], "MB session out"=w306:refnum<class "MB_Master.lvclass">)  [unwired: 5 in]
            n183 = global write "采配水全局变量.vi" "报警簇"(w326) -> ()
          }
          frame "读参数" {
            n184 = call <vilib>:"Read Holding Registers.vi"("error in (no error)"=w358, "quantity"=u16 24 ("number of holding registers"), "starting address"=u16 100, "MB session in"=w359) -> ("error out"=w353:errorcluster, "Registers"=w355:u16[], "MB session out"=w354:refnum<class "MB_Master.lvclass">)  [unwired: 5 in]
            n185 = Array To Cluster(array=w355) -> (cluster=w352:T20)
            n186 = global write "采配水全局变量.vi" "参数设置"(w352) -> ()
          }
          frame "多个写入" {
            n187 = Unbundle By Name(w365) -> ("数据"=w364:variant)
            n188 = Variant To Data(type=T14 {"starting address"=0, "holding register values"=[]}, Variant=w364) -> (data=w362:T14)  [unwired: 1 in, 1 out]
            n189 = Unbundle By Name(w362) -> ("starting address"=w361:u16, "holding register values"=w360:u16[])
            n190 = call <vilib>:"Write Multiple Registers.vi"("error in (no error)"=w368, "values"=w360, "starting address"=w361, "MB session in"=w369) -> ("error out"=w367:errorcluster, "MB session out"=w366:refnum<class "MB_Master.lvclass">)  [unwired: 6 in]
          }
          frame "单个写入" {
            n191 = Unbundle By Name(w375) -> ("数据"=w374:variant)
            n192 = Variant To Data(type=T15 {"starting address"=0, "holding register value"=0}, Variant=w374) -> (data=w372:T15)  [unwired: 1 in, 1 out]
            n193 = Unbundle By Name(w372) -> ("starting address"=w371:u16, "holding register value"=w370:u16)
            n194 = call <vilib>:"Write Single Register.vi"("error in (no error)"=w378, "value"=w370, "address"=w371, "MB session in"=w379) -> ("error out"=w377:errorcluster, "MB session out"=w376:refnum<class "MB_Master.lvclass">)  [unwired: 6 in]
          }
          frame "线圈写入" {
            n195 = Unbundle By Name(w385) -> ("数据"=w384:variant)
            n196 = Variant To Data(type=T16 {"starting address"=0, "coil values"=[]}, Variant=w384) -> (data=w382:T16)  [unwired: 1 in, 1 out]
            n197 = Unbundle By Name(w382) -> ("starting address"=w381:u16, "coil values"=w380:bool[])
            n198 = call <vilib>:"Write Multiple Coils.vi"("error in (no error)"=w388, "values"=w380, "starting address"=w381, "MB session in"=w389) -> ("error out"=w387:errorcluster, "MB session out"=w386:refnum<class "MB_Master.lvclass">)  [unwired: 6 in]
          }
          frame "shutdown" {
            n199 = call <vilib>:"Write Single Register.vi"("error in (no error)"=w395, "value"=u16 0, "address"=u16 4047, "MB session in"=w399) -> ("error out"=w394:errorcluster, "MB session out"=w398:refnum<class "MB_Master.lvclass">)  [unwired: 6 in]
            n200 = call-dynamic "Close Session.vi"("error in (no error)"=w394, "MB session in"=w398) -> ("error out"=w400:errorcluster)  [unwired: 9 in]
            n201 = call "文件对话框"("start path"=path "D:/SRC") -> ("selected path"=w393:path, "cancelled"=w391:bool)  [unwired: 11 in, 2 out]
            n202 = call <vilib>:"Clear Errors.vi"("error in (no error)"=w400) -> ("error out"=w390:errorcluster)  [unwired: 5 in, 1 out]
            n203 = case shown="假" w391 {
              tunnel: w393 -> [w406 _]
              tunnel: w390 -> [_ _]
              frame False {
                n204 = Path To String(path=w406) -> (string=w403:string)
                n205 = Format Into String(format string="  - \"%s\"" ("格式字符串"), initial string="\"C:\\Program Files\\Fatek\\WinProladder\\WProlad.exe\"" ("command line"), w403) -> (resulting string=w404:string)  [unwired: 1 in, 1 out]
                n206 = call <vilib>:"System Exec.vi"("command line"=w404) -> ("error out"=w407:errorcluster)  [unwired: 7 in, 3 out]
                n207 = case shown="错误" w407 {
                  tunnel: w403 -> [_ w410]
                  frame No Error {
                  }
                  frame Error {
                    n208 = Format Into String(format string="  - \"%s\"" ("格式字符串"), initial string="\"C:\\Program Files (x86)\\Fatek\\WinProladder\\WProlad.exe\"" ("command line"), w410) -> (resulting string=w408:string)  [unwired: 1 in, 1 out]
                    n209 = call <vilib>:"System Exec.vi"("command line"=w408) -> ()  [unwired: 7 in, 4 out]
                  }
                }
              }
              frame True {
              }
            }
          }
        }
      }
      frame Error {
        n210 = property class="MB_Master"(reference=w413) -> (reference out=w412:refnum<class "MB_Master.lvclass">, "Properties:Session Valid"=w414:bool)  [unwired: 1 in, 1 out]
        n211 = Flush Queue(queue=w419) -> (queue out=w418:refnum<queue>)  [unwired: 1 in, 2 out]
        n212 = Wait (ms)(milliseconds to wait=u32 2000 ("等待时间（毫秒）")) -> ()  [unwired: 1 out]
        n213 = case shown="假" w414 {
          tunnel: w418 -> [w421 _]
          frame False {
            n214 = Enqueue Element At Opposite End(queue=w421, element=cluster{"命令":string, "数据":variant} {"命令"="init", "数据"=variant} ("元素")) -> ()  [unwired: 2 in, 3 out]
          }
          frame True {
          }
        }
        n215 = call <vilib>:"Clear Errors.vi"("error in (no error)"=w415) -> ("error out"=w416:errorcluster)  [unwired: 5 in, 1 out]
      }
    }
    n216 = Unbundle By Name(w278) -> ("status"=→"通讯故障":bool)
  }
  n217 = property on="多列列表框" class="MCListbox (严格)"("ItemNames"=string[][] [["待机"], ["初始化"], ["流通池润洗"], ["沉淀池润洗"], ["采样"], ["沉淀"], ["配水"], ["外部管路反冲洗"], ["内部管路反冲洗"], ["流通池储水"], ["结束"]] ("项名")) -> ()  [unwired: 2 in, 2 out]
  n218 = call-dynamic "Close Session.vi"("error in (no error)"=w1, "MB session in"=w4) -> ()  [unwired: 9 in, 1 out]
